vi "Get Shared Library Name.vi"(8 "error in (no error)":errorcluster, 11 "DLL in":refnum<class "NI_AB_API_DLL.lvclass">) -> (0 "error out":errorcluster, 2 "Shared library file name":string, 3 "DLL out":refnum<class "NI_AB_API_DLL.lvclass">)   [LabVIEW 2020, in "NI_AB_API_DLL.lvclass"]
uses:
  <vilib>/AppBuilder/AB_API/DLL/NI_AB_API_DLL.lvclass
  e:/builds/penguin/labview/branches/2020/dev/dist/vi.lib/AppBuilder/AB_API/Build/NI_AB_API_Build.lvclass
  <vilib>/AppBuilder/AB_Classes/TargetFile/AB_Targetfile.lvclass
  <vilib>/AppBuilder/AB_API/Build/NI_AB_API_Build.lvclass
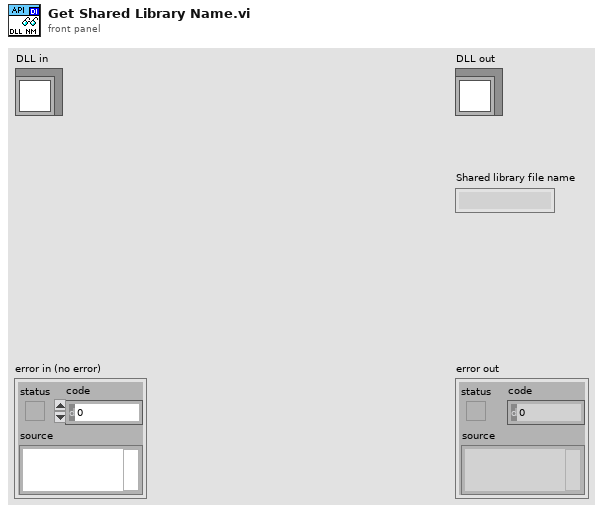
[diagram p1: front panel]
types:
  T1 = typedef "AB_Targetfile.ctl" = cluster{"targetfileName":string, "targetfileGUID":string, "enableDebugging":bool, "versionInfo":cluster{"productName":string, "legalCopyright":string, "companyName":string, "internalName":string, "fileDescription":string}, "eng_consolidatedTypeInfo":string, "fastFileFormat":bool, "eng_LEIFBuildData":u32, "versionIndependent":bool}
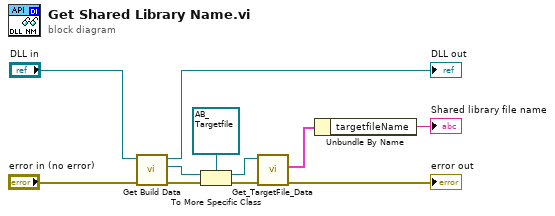
[diagram p0: block diagram]
diagram:
  n1 = call <vilib>:"Get Build Data.vi"("error in (no error)"="error in (no error)", "NI_AB_API_Build in"="DLL in") -> ("error out"=w8:errorcluster, "AB_Build.lvclass"=w7:refnum<class "AB_Build.lvclass">, "NI_AB_API_Build out"=→"DLL out":refnum<class "NI_AB_API_DLL.lvclass">)  [unwired: 7 in]
  n2 = To More Specific Class(target class=refnum<class "AB_Targetfile.lvclass"> refnum ("AB_Targetfile.lvclass"), reference=w7, error in=w8) -> (specific class reference=w1:refnum<class "AB_Targetfile.lvclass">, error out=w4:errorcluster)
  n3 = call <vilib>:"Get_TargetFile_Data.vi"("error in (no error)"=w4, "AB_Targetfile in"=w1) -> ("error out"=→"error out":errorcluster, "data"=w5:T1)  [unwired: 7 in, 1 out]
  n4 = Unbundle By Name(w5) -> ("targetfileName"=→"Shared library file name":string)
